vi "Timer.vi"() -> ()   [LabVIEW 2015]
panel:
  in  "stop 5":bool
  in  "stop 2":bool
  out "Numeric":dbl
  in  "Tab Control":enum32{"Page 1", "Page 2"}(tab)
  out "Hours":dbl
  out "Minutes":dbl
  out "Second":dbl
  in  "stop":bool
  in  "Play Button":bool
  in  "Blinking Mode ON":bool
  in  "Tab Control 2":enum32{"Page 1", "Page 2"}(tab)
  out "Boolean 9":bool
  out "Boolean 10":bool
  in  "Up Button":bool
  in  "?":bool
  out "Boolean 8":bool
  out "Boolean 6":bool
  out "Boolean":bool
  out "Boolean 7":bool
  in  "?":bool
  in  "?":bool
  out "Boolean 5":bool
  in  "Water Quantity":bool
  out "Filter Water":dbl(slide)
  in  "Electric Owan Fix\n Heating range":dbl(slide) scale=0.0..25.0
  out "Boolean 3":bool
  out "Boolean 4":bool
  out "?":dbl(slide) scale=0.0..100.0
  out "Boolean 2":bool
  in  "Start":bool
  in  "Water Quantity 2":bool
  out "Milk":dbl(slide) scale=0.0..100.0
  out "Milk enter in tank":dbl
  in  "stop 3":bool
  out "Sugar/Chini":dbl(slide) scale=0.0..100.0
  out "Filter Water  2":dbl(slide) scale=0.0..100.0
  in  "stop 4":bool
  in  "Up Button 2":bool
  out "s? t:f":dbl
  out "s? t:f 2":dbl
  out "Water Status":string
  in  "?":bool
  out "Numeric 2":dbl
  out "?":dbl
  # "Smart Programming Real Time Watch"
  # "Tea Recipe"
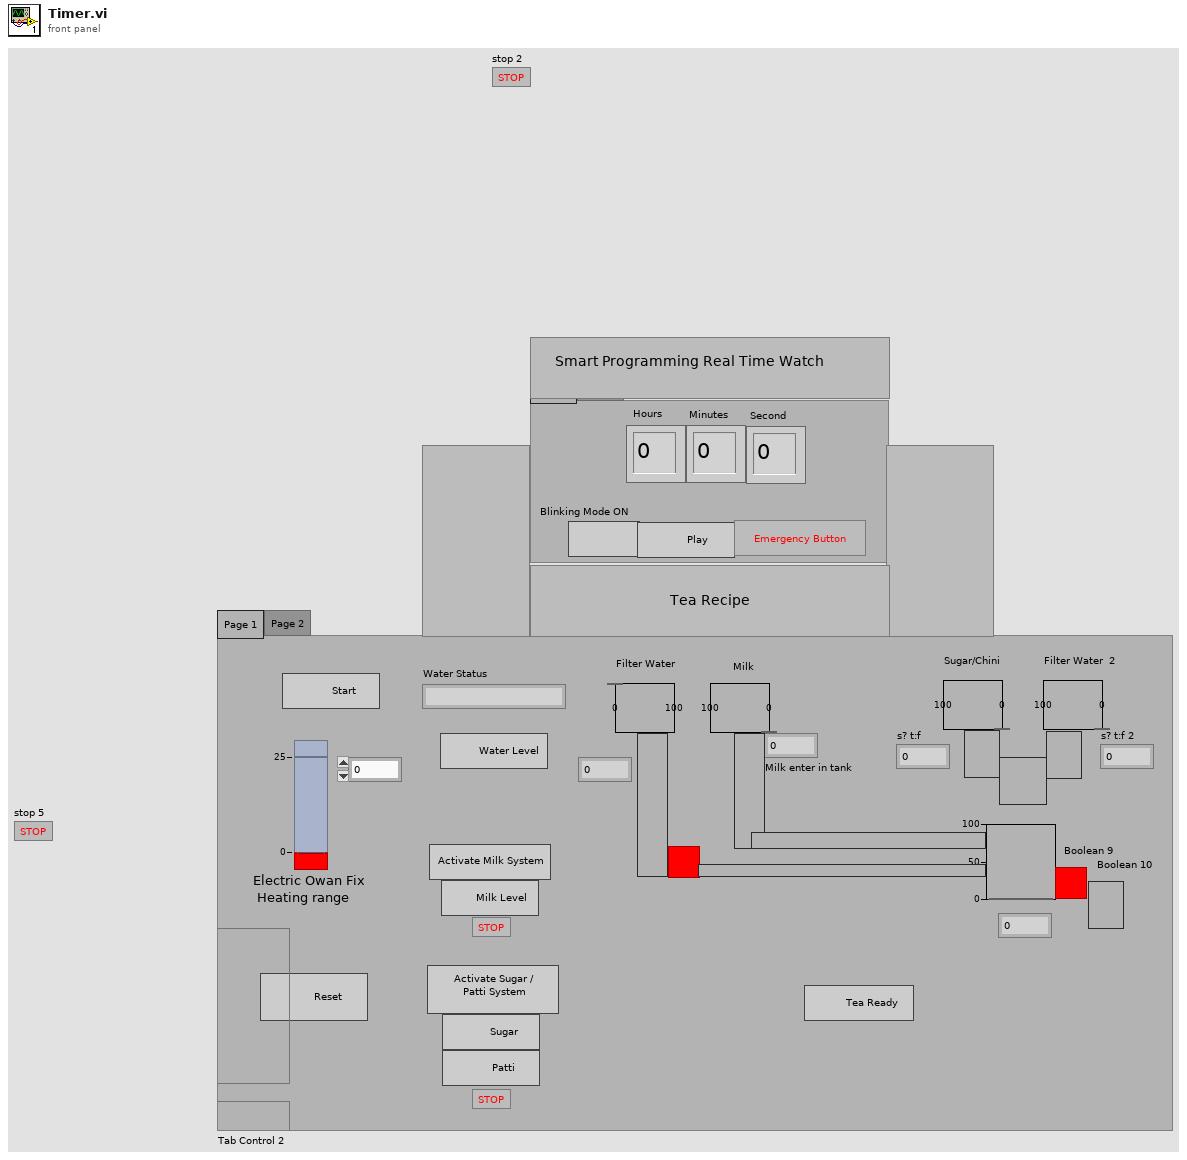
[diagram p1: front panel]
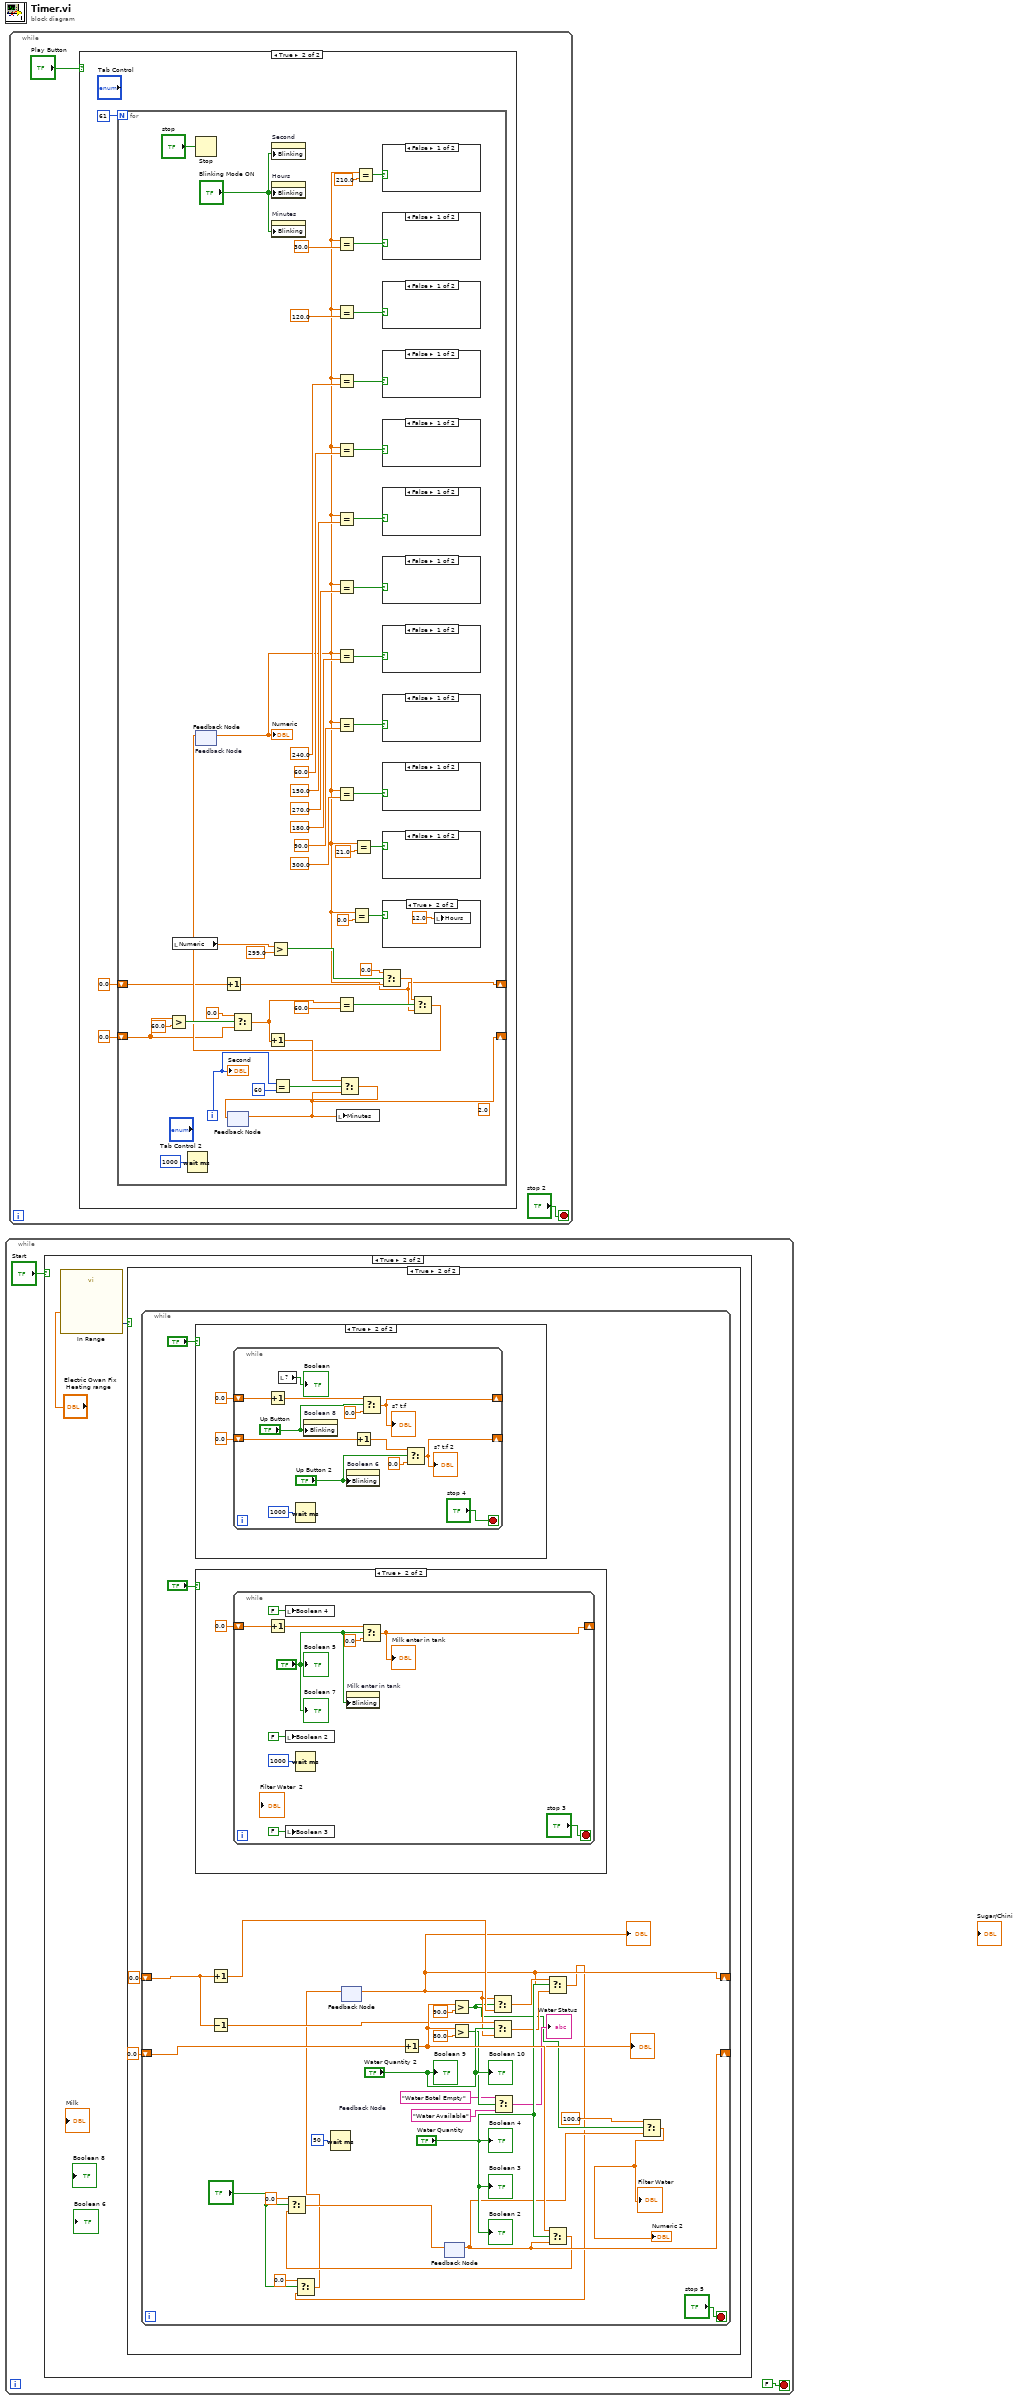
[diagram p0: block diagram]
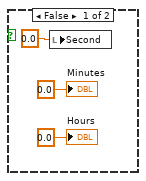
[diagram p2: hidden frame]
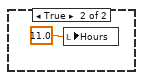
[diagram p4: hidden frame]
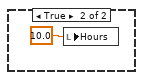
[diagram p5: hidden frame]
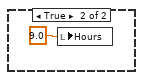
[diagram p6: hidden frame]
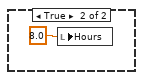
[diagram p7: hidden frame]
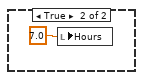
[diagram p8: hidden frame]
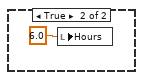
[diagram p9: hidden frame]
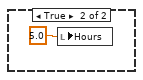
[diagram p10: hidden frame]
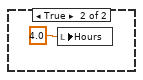
[diagram p11: hidden frame]
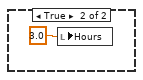
[diagram p12: hidden frame]
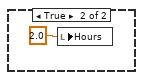
[diagram p13: hidden frame]
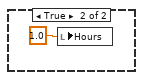
[diagram p14: hidden frame]
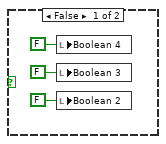
[diagram p16: hidden frame]
diagram:
  n1 = while {
    stop <- FALSE stop-if-true
    n2 = case shown="True" "Start" {
      frame False {
      }
      frame True {
        n3 = call "In Range"("Operand 1"="Electric Owan Fix\n Heating range") -> ("Result"=w3:dynamicdata)  [unwired: 9 in, 1 out]
        n4 = case shown="True" w3 {
          frame False {
            n5 = local write "Boolean 4"(FALSE ("Boolean 4")) -> ()
            n6 = local write "Boolean 3"(FALSE ("Boolean 3")) -> ()
            n7 = local write "Boolean 2"(FALSE ("Boolean 2")) -> ()
          }
          frame True {
            n8 = while {
              shift-right: [w21] -> _
              shift-left: 0.0 -> [w23]
              shift-right: [w19] -> _
              shift-left: 0.0 -> [w22]
              stop <- "stop 5" stop-if-true
              n9 = case shown="True" "?" {
                frame False {
                }
                frame True {
                  n10 = while {
                    shift-right: [w53] -> _
                    shift-left: 0.0 -> [w52]
                    shift-right: [w45] -> _
                    shift-left: 0.0 -> [w47]
                    stop <- "stop 4" stop-if-true
                    n11 = Increment(x=w52) -> (x+1=w54:dbl)
                    n12 = local read item#31() -> (→"Boolean":bool)
                    n13 = Wait (ms)(milliseconds to wait=u32 1000) -> ()  [unwired: 1 out]
                    n14 = property on="Boolean 8" class="Bool (strict)"("Blinking"="Up Button") -> ()  [unwired: 2 in, 2 out]
                    n15 = property on="Boolean 6" class="Bool (strict)"("Blinking"="Up Button 2") -> ()  [unwired: 2 in, 2 out]
                    n16 = Increment(x=w47) -> (x+1=w48:dbl)
                    n17 = Select(t=w54, s="Up Button", f=0.0) -> (s? t:f=w53:dbl)
                    "s? t:f" <- w53
                    n18 = Select(t=w48, s="Up Button 2", f=0.0) -> (s? t:f=w45:dbl)
                    "s? t:f 2" <- w45
                  }
                }
              }
              n19 = case shown="True" "?" {
                frame False {
                }
                frame True {
                  n20 = while {
                    shift-right: [w64] -> _
                    shift-left: 0.0 -> [w65]
                    stop <- "stop 3" stop-if-true
                    n21 = Increment(x=w65) -> (x+1=w66:dbl)
                    n22 = local write "Boolean 4"(FALSE ("Boolean 4")) -> ()
                    n23 = local write "Boolean 2"(FALSE ("Boolean 2")) -> ()
                    n24 = local write "Boolean 3"(FALSE ("Boolean 3")) -> ()
                    n25 = Wait (ms)(milliseconds to wait=u32 1000) -> ()  [unwired: 1 out]
                    n26 = property on="Milk enter in tank" class="DigNum (strict)"("Blinking"="?") -> ()  [unwired: 2 in, 2 out]
                    n27 = Select(t=w66, s="?", f=0.0) -> (s? t:f=w64:dbl)
                    "Milk enter in tank" <- w64
                    "Boolean 5" <- "?"
                    "Boolean 7" <- "?"
                  }
                }
              }
              n28 = Increment(x=w23) -> (x+1=w35:dbl)
              n29 = Decrement(x=w23) -> (x-1=w26:dbl)
              n30 = Wait (ms)(milliseconds to wait=u32 50) -> ()  [unwired: 1 out]
              n31 = feedback #1() -> (w21:dbl)  [unwired: 1 in]
              "?" <- w21
              "?" <- w21
              n32 = Increment(x=w22) -> (x+1=w37:dbl)
              n33 = feedback #2() -> (w19:dbl)  [unwired: 1 in]
              n34 = Greater?(x=w37, y=90.0) -> (0:w20:bool)
              n35 = Greater?(x=w37, y=80.0) -> (0:w29:bool)
              n36 = Select(t=w21, s=w20, f=w35) -> (s? t:f=w36:dbl)
              n37 = Select(t=w26, s="Water Quantity 2", f=w21) -> (s? t:f=w27:dbl)
              n38 = Select(t="Water Botel Empty", s=w29, f="Water Available") -> (s? t:f=→"Water Status":string)
              n39 = Select(t=w36, s="Water Quantity", f=w27) -> (s? t:f=w10:dbl)
              n40 = Select(t=0.0, s="?", f=w10) -> (s? t:f=w11:dbl)
              n41 = feedback-in #1(w11) -> ()
              n42 = Select(t=w37, s="Water Quantity", f=w19) -> (s? t:f=w14:dbl)
              n43 = Select(t=0.0, s="?", f=w14) -> (s? t:f=w15:dbl)
              n44 = feedback-in #2(w15) -> ()
              n45 = Select(t=100.0, s=w20, f=w19) -> (s? t:f=→"Filter Water" →"Numeric 2":dbl)
              "Boolean 2" <- "Water Quantity"
              "Boolean 4" <- "Water Quantity"
              "Boolean 3" <- "Water Quantity"
              "Boolean 10" <- "Water Quantity 2"
              "Boolean 9" <- "Water Quantity 2"
            }
          }
        }
      }
    }
  }
  n46 = while {
    stop <- "stop 2" stop-if-true
    n47 = case shown="True" "Play Button" {
      frame False {
        n48 = local write "Second"(0.0 ("Second")) -> ()
        "Hours" <- 0.0 ("Hours")
        "Minutes" <- 0.0 ("Minute")
      }
      frame True {
        n49 = for {
          N: 61 -> [_]
          shift-right: [w78] -> _
          shift-left: 0.0 -> [w113]
          shift-right: [w79] -> _
          shift-left: 0.0 -> [w96]
          i -> [w123]
          (unwired) 2.0 ("x")
          n50 = Greater?(x=w113, y=60.0) -> (0:w118:bool)
          n51 = local read "Numeric"() -> (w99:dbl)
          n52 = Wait (ms)(milliseconds to wait=u32 1000) -> ()  [unwired: 1 out]
          n53 = Stop(stop? (T)="stop") -> ()
          n54 = feedback #3 "Feedback Node"() -> (w79:dbl)  [unwired: 1 in]
          "Numeric" <- w79
          n55 = Increment(x=w96) -> (x+1=w95:dbl)
          n56 = feedback #4 "Feedback Node"() -> (w78:dbl)  [unwired: 1 in]
          n57 = Select(t=0.0, s=w118, f=w113) -> (s? t:f=w111:dbl)
          n58 = Increment(x=w111) -> (x+1=w120:dbl)
          n59 = Greater?(x=w99, y=299.0) -> (0:w98:bool)
          n60 = property on="Second" class="DigNum (strict)"("Blinking"="Blinking Mode ON") -> ()  [unwired: 2 in, 2 out]
          n61 = property on="Hours" class="DigNum (strict)"("Blinking"="Blinking Mode ON") -> ()  [unwired: 2 in, 2 out]
          n62 = property on="Minutes" class="DigNum (strict)"("Blinking"="Blinking Mode ON") -> ()  [unwired: 2 in, 2 out]
          n63 = Equal?(x=w123, y=60) -> (x = y?=w121:bool)
          n64 = Equal?(x=w79, y=30.0) -> (x = y?=w109:bool)
          n65 = Equal?(x=w79, y=120.0) -> (x = y?=w101:bool)
          n66 = Equal?(x=w79, y=240.0) -> (x = y?=w85:bool)
          n67 = Equal?(x=w79, y=60.0) -> (x = y?=w107:bool)
          n68 = Equal?(x=w79, y=150.0) -> (x = y?=w102:bool)
          n69 = Equal?(x=w79, y=270.0) -> (x = y?=w84:bool)
          n70 = Equal?(x=w79, y=180.0) -> (x = y?=w81:bool)
          n71 = Equal?(x=w79, y=90.0) -> (x = y?=w105:bool)
          n72 = Equal?(x=w79, y=300.0) -> (x = y?=w83:bool)
          n73 = Equal?(x=w111, y=60.0) -> (x = y?=w112:bool)
          n74 = local write "Minutes"(w78) -> ()
          n75 = Select(t=w120, s=w121, f=w78) -> (s? t:f=w119:dbl)
          n76 = feedback-in #4(w119) -> ()
          n77 = Equal?(x=w79, y=0.0) -> (x = y?=w82:bool)
          n78 = Equal?(x=w79, y=21.0) -> (x = y?=w80:bool)
          n79 = Equal?(x=w79, y=210.0) -> (x = y?=w86:bool)
          n80 = Select(t=0.0, s=w98, f=w95) -> (s? t:f=w94:dbl)
          n81 = case shown="False" w86 {
            frame False {
            }
            frame True {
              n82 = local write "Hours"(8.0 ("Hours")) -> ()
            }
          }
          n83 = case shown="False" w109 {
            frame False {
            }
            frame True {
              n84 = local write "Hours"(1.0 ("Hours")) -> ()
            }
          }
          n85 = case shown="False" w101 {
            frame False {
            }
            frame True {
              n86 = local write "Hours"(4.0 ("Hours")) -> ()
            }
          }
          n87 = case shown="False" w85 {
            frame False {
            }
            frame True {
              n88 = local write "Hours"(9.0 ("Hours")) -> ()
            }
          }
          n89 = case shown="False" w107 {
            frame False {
            }
            frame True {
              n90 = local write "Hours"(2.0 ("Hours")) -> ()
            }
          }
          n91 = case shown="False" w102 {
            frame False {
            }
            frame True {
              n92 = local write "Hours"(5.0 ("Hours")) -> ()
            }
          }
          n93 = case shown="False" w84 {
            frame False {
            }
            frame True {
              n94 = local write "Hours"(10.0 ("Hours")) -> ()
            }
          }
          n95 = case shown="False" w81 {
            frame False {
            }
            frame True {
              n96 = local write "Hours"(6.0 ("Hours")) -> ()
            }
          }
          n97 = case shown="False" w105 {
            frame False {
            }
            frame True {
              n98 = local write "Hours"(3.0 ("Minute")) -> ()
            }
          }
          n99 = case shown="False" w83 {
            frame False {
            }
            frame True {
              n100 = local write "Hours"(11.0 ("Hours")) -> ()
            }
          }
          n101 = case shown="False" w80 {
            frame False {
            }
            frame True {
              n102 = local write "Hours"(7.0 ("Hours")) -> ()
            }
          }
          n103 = case shown="True" w82 {
            frame False {
            }
            frame True {
              n104 = local write "Hours"(12.0 ("Hours")) -> ()
            }
          }
          n105 = Select(t=w94, s=w112, f=w79) -> (s? t:f=w114:dbl)
          n106 = feedback-in #3(w114) -> ()
          "Second" <- w123
        }
      }
    }
  }
